vi "MemoryOperationCopy.vi"(6 "DestinationPath":string, 7 "DestinationPathBufferSize":i32=2048 caption="DestinationPathBufferSize (2048)", 8 "error in (no error)":errorcluster {"code" format="%.0x"}, 9 "SourcePath":string, 10 "SourcePathBufferSize":i32=2048 caption="SourcePathBufferSize (2048)", 11 "instrument handle":refnum<k15>) -> (0 "error out":errorcluster {"code" format="%.0x"}, 3 "instrument handle out":refnum<k15>)   [LabVIEW 2009, in "Keysight XSAn.lvlib"]
doc: "Copies an existing file to a new file or an existing directory to a new directory.\n\nSupported Models: All supported"
uses:
  <instrlib>/Keysight XSAn/Keysight XSAn.lvlib
  AgXSAn.dll
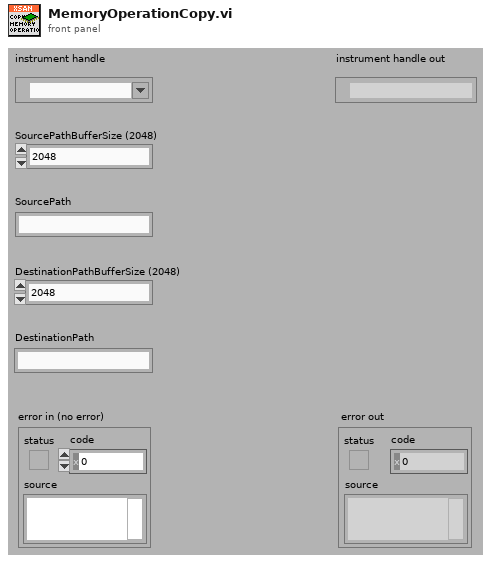
[diagram p1: front panel]
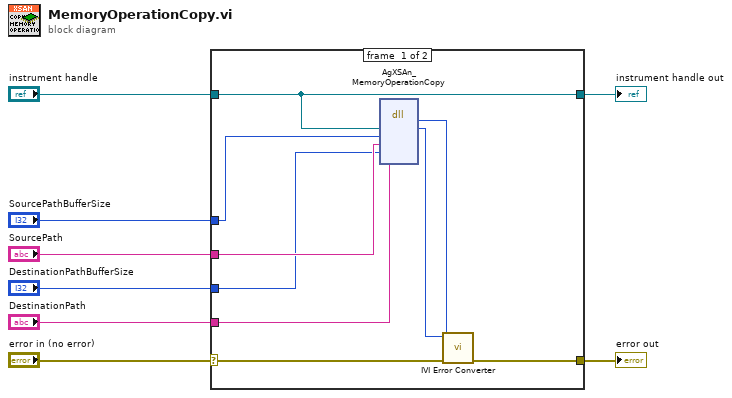
[diagram p0: block diagram]
diagram:
  n1 = case shown="No Error" "error in (no error)" {
    selector: "error in (no error)" -> [w15 w19]
    tunnel: [w14 w19] -> w8
    tunnel: "instrument handle" -> [w9 w18]
    tunnel: "SourcePathBufferSize" -> [w13 _]
    tunnel: "SourcePath" -> [w12 _]
    tunnel: "DestinationPathBufferSize" -> [w11 _]
    tunnel: "DestinationPath" -> [w10 _]
    tunnel: [w9 w18] -> w1
    frame #0 {
      n2 = dll-call lib="AgXSAn**.dll" fn="AgXSAn_MemoryOperationCopy"("Vi"=w9, "SourcePathBufferSize"=w13, "SourcePath"=w12, "DestinationPathBufferSize"=w11, "DestinationPath"=w10) -> (w16:i32, "Vi"=w17:u32)  [unwired: 7 in, 2 out]
      n3 = call <instrlib>:"IVI Error Converter.vi"("error in (no error)"=w15, "IVI error code (0)"=w16, "instrument handle"=w17) -> ("error out"=w14:errorcluster)  [unwired: 7 in, 1 out]
    }
    frame #1 {
    }
  }
  "error out" <- w8
  "instrument handle out" <- w1
